vi "roboRIO v1.0 Build MUX Configuration Accelerometer.vi"(11 "Accelerometer Channels List":T4) -> (3 "Channel Reservation Info":T1)   [LabVIEW 2021]
uses:
  <vilib>/myRIO/Common/Instrument Driver Framework/myRIO v1.0/Accelerometer/typedefs/Accelerometer Channels List.ctl
  <vilib>/myRIO/Common/Instrument Driver Framework/myRIO v1.0/Accelerometer/typedefs/Accelerometer Channels Enum.ctl
  <vilib>/myRIO/Common/Instrument Driver Framework/roboRIO v1.0/Resource Manager/typedefs/roboRIO v1.0 Channel Reservation List.ctl
  <vilib>/myRIO/Common/Instrument Driver Framework/roboRIO v1.0/Resource Manager/typedefs/roboRIO v1.0 Channel Reservation Info.ctl
  <vilib>/myRIO/Common/Instrument Driver Framework/roboRIO v1.0/Resource Manager/typedefs/roboRIO v1.0 Connector List.ctl
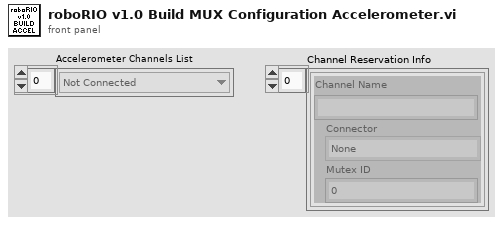
[diagram p1: front panel]
types:
  T1 = typedef "roboRIO v1.0 Channel Reservation List.ctl" = T2[]
  T2 = typedef "roboRIO v1.0 Channel Reservation Info.ctl" = cluster{"Channel Name":string, "Connector":T3, "Mutex ID":i32}
  T3 = typedef "roboRIO v1.0 Connector List.ctl" = enum32{"None", "ConnectorB", "ConnectorI2C", "ConnectorDIO", "ConnectorRSL", "ConnectorRELAY", "ConnectorAI", "ConnectorPWM", "ConnectorSPI"}
  T4 = typedef "Accelerometer Channels List.ctl" = T5[]
  T5 = typedef "Accelerometer Channels Enum.ctl" = enum16{"Not Connected", "X-Axis", "Y-Axis", "Z-Axis"}
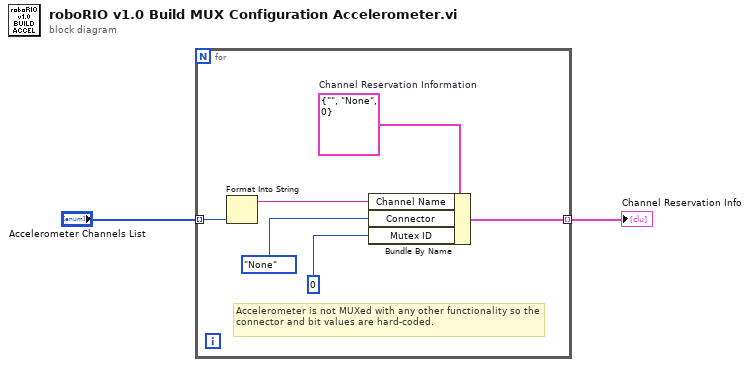
[diagram p0: block diagram]
diagram:
  n1 = for {
    tunnel: "Accelerometer Channels List" -> [w8] mode=indexing
    tunnel: [w3] -> w1 mode=indexing
    w7 = T2 {"Channel Name"="", "Connector"=enum."None", "Mutex ID"=0}  # Channel Reservation Information
    # "Accelerometer is not MUXed with any other functionality so the connector and bit values are hard-coded."
    n2 = Format Into String(w8) -> (resulting string=w6:string)  [unwired: 3 in, 1 out]
    n3 = Bundle By Name(cluster=w7, "Channel Name"=w6, "Connector"=roboRIO_v1.0_Connector_List."None", "Mutex ID"=0 ("Bit")) -> (w3:T2)
  }
  "Channel Reservation Info" <- w1
